vi "Register Groups.vi"(8 "error in (no error)":errorcluster, 10 "Groups":refnum<class "Group.lvclass">[](array[class]), 11 "DataHandlerAPI in":refnum<class "DataHandlerAPI.lvclass">) -> (0 "error out":errorcluster, 3 "DataHandlerAPI out":refnum<class "DataHandlerAPI.lvclass">)   [LabVIEW 2020, in "Volatus.lvlib" / "DataHandlerAPI.lvclass"]
uses:
  DataHandlerAPI.lvclass
  lv-vecto/Vecto/Group/Group.lvclass
  DataHandlerAPI.lvclass/DataHandlerAPI.ctl
  DataHandler Messages/Register Groups Msg/Register Groups Msg.lvclass
  lv-promises/Promises/Promise/Promise.lvclass
  lv-promises/Promises/Error Result/Error Result.lvclass
  lv-promises/Promises/Future/Future.lvclass
  C:/dev/lv20CE/relink/lv-promises/Promises/Value/Value.lvclass
  C:/dev/lv20CE/relink/lv-promises/Promises/Error Result/Error Result.lvclass
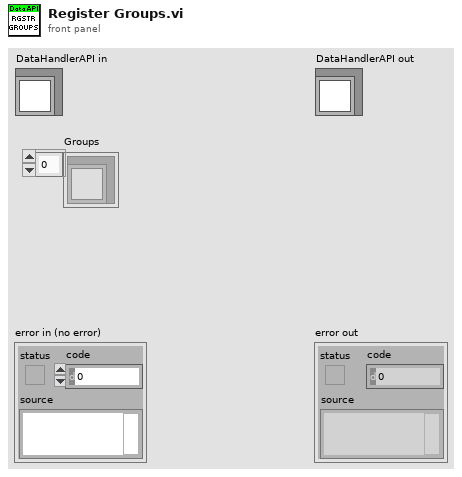
[diagram p1: front panel]
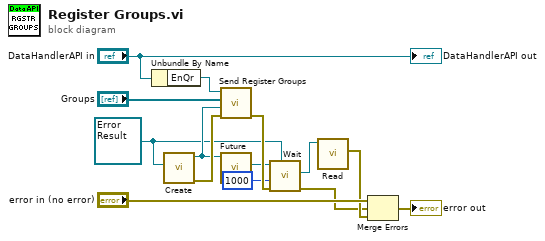
[diagram p0: block diagram]
diagram:
  w6 = refnum<class "Error Result.lvclass"> refnum ("Futures:Error Result.lvclass")
  n1 = Unbundle By Name("DataHandlerAPI in") -> ("EnQr"=w11:refnum<class "Message Enqueuer.lvclass">)
  n2 = call "Create.vi"("Result Type"=w6) -> ("error out"=w9:errorcluster, "Promise"=w8:refnum<class "Promise.lvclass">)  [unwired: 9 in]
  n3 = call "Send Register Groups.vi"("error in (no error)"=w9, "Promise"=w8, "Groups"="Groups", "Message Enqueuer"=w11) -> ("error out"=w14:errorcluster)  [unwired: 6 in, 1 out]
  n4 = call "Future.vi"("Promise in"=w8) -> ("Future"=w7:refnum<class "Future.lvclass">)  [unwired: 9 in, 1 out]
  n5 = call "Wait.vi"("Result Type"=w6, "error in (no error)"=w14, "Timeout mS (-1)"=1000, "Future in"=w7) -> ("error out"=w1:errorcluster, "Result"=w4:refnum<class "Error Result.lvclass">)  [unwired: 6 in]
  n6 = call "Read.vi"("Error Result in"=w4) -> ("Error"=w2:errorcluster)  [unwired: 10 in]
  n7 = Merge Errors("error in (no error)", w1, w2) -> (→"error out":errorcluster)
  "DataHandlerAPI out" <- "DataHandlerAPI in"
